vi "VI4.vi"() -> ()   [LabVIEW 2010]
panel:
  in  "AS_RS Ativado":bool
  in  "Elevar Z":bool
  in  "ARMAZEM_PEGAR":bool
  in  "ESTEIRA_PEGAR":bool
  out "YD3":dbl
  out "YD2":dbl
  out "YD1":dbl
  out "YD0":dbl
  in  "Coordenada_Y":dbl min=0.0 max=2.0
  out "Z_Pos_Ok":bool
  out "Y_Pos_Ok":bool
  out "X_Pos_Ok":bool
  out "Z_Home_Ok":bool
  out "Y_Home_Ok":bool
  out "X_Home_Ok":bool
  in  "Z_CTRG":bool
  in  "Y_CTRG":bool
  in  "X_CTRG":bool
  in  "Z_HOME":bool
  in  "Y_HOME":bool
  in  "X_HOME":bool
  in  "Start":bool
  in  "Confirmação da posição":bool
  out "ZD3":dbl
  out "ZD2":dbl
  out "ZD1":dbl
  out "ZD0":dbl
  out "XD3":dbl
  out "XD2":dbl
  out "XD1":dbl
  out "XD0":dbl
  in  "Coordenada_Z":dbl min=0.0 max=12.0
  in  "Coordenada_X":dbl min=0.0 max=6.0
  out "Esteira 4":bool
  out "Esteira 3":bool
  out "Esteira 2":bool
  out "Esteira 1":bool
  in  "Eletroválvula 4":bool
  in  "Eletroválvula 3":bool
  in  "Eletroválvula 2":bool
  in  "Eletroválvula 1":bool
  out "Sensor 4":bool
  out "Sensor 3":bool
  out "Sensor 2":bool
  out "Sensor 1":bool
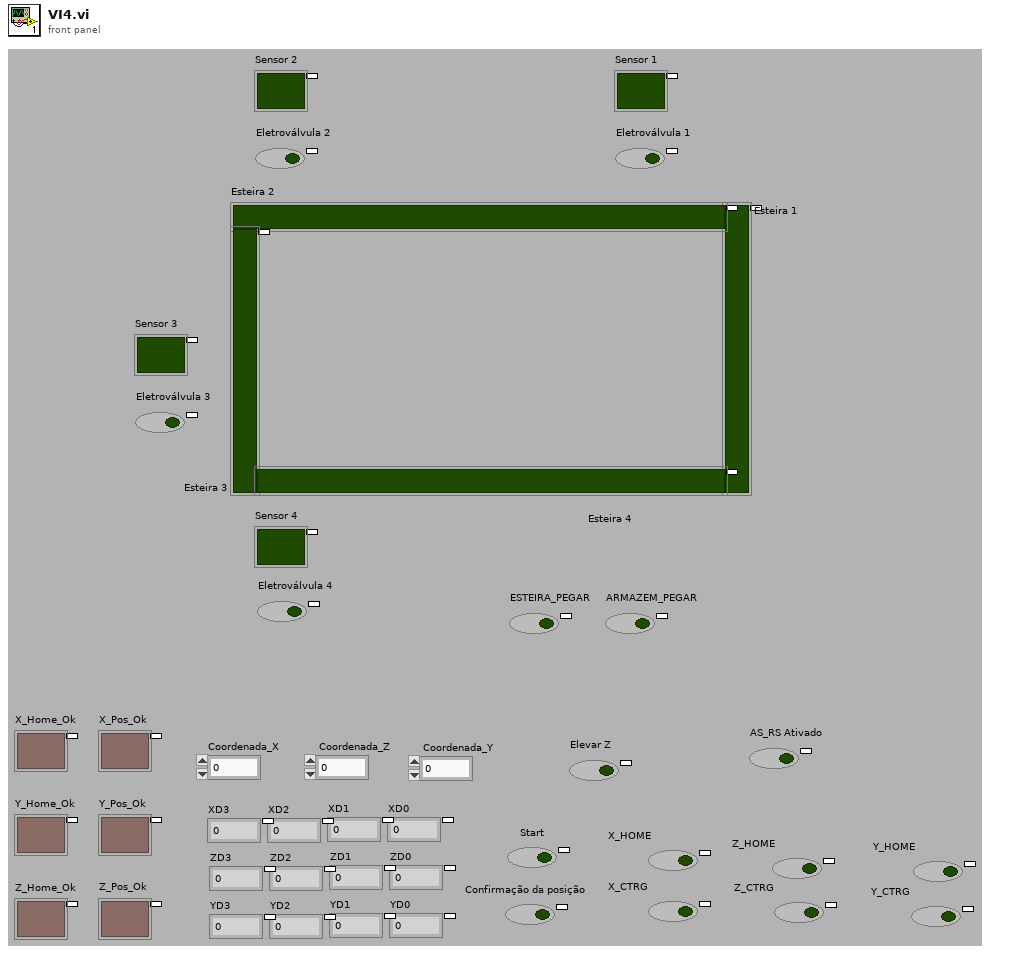
[diagram p1: front panel]
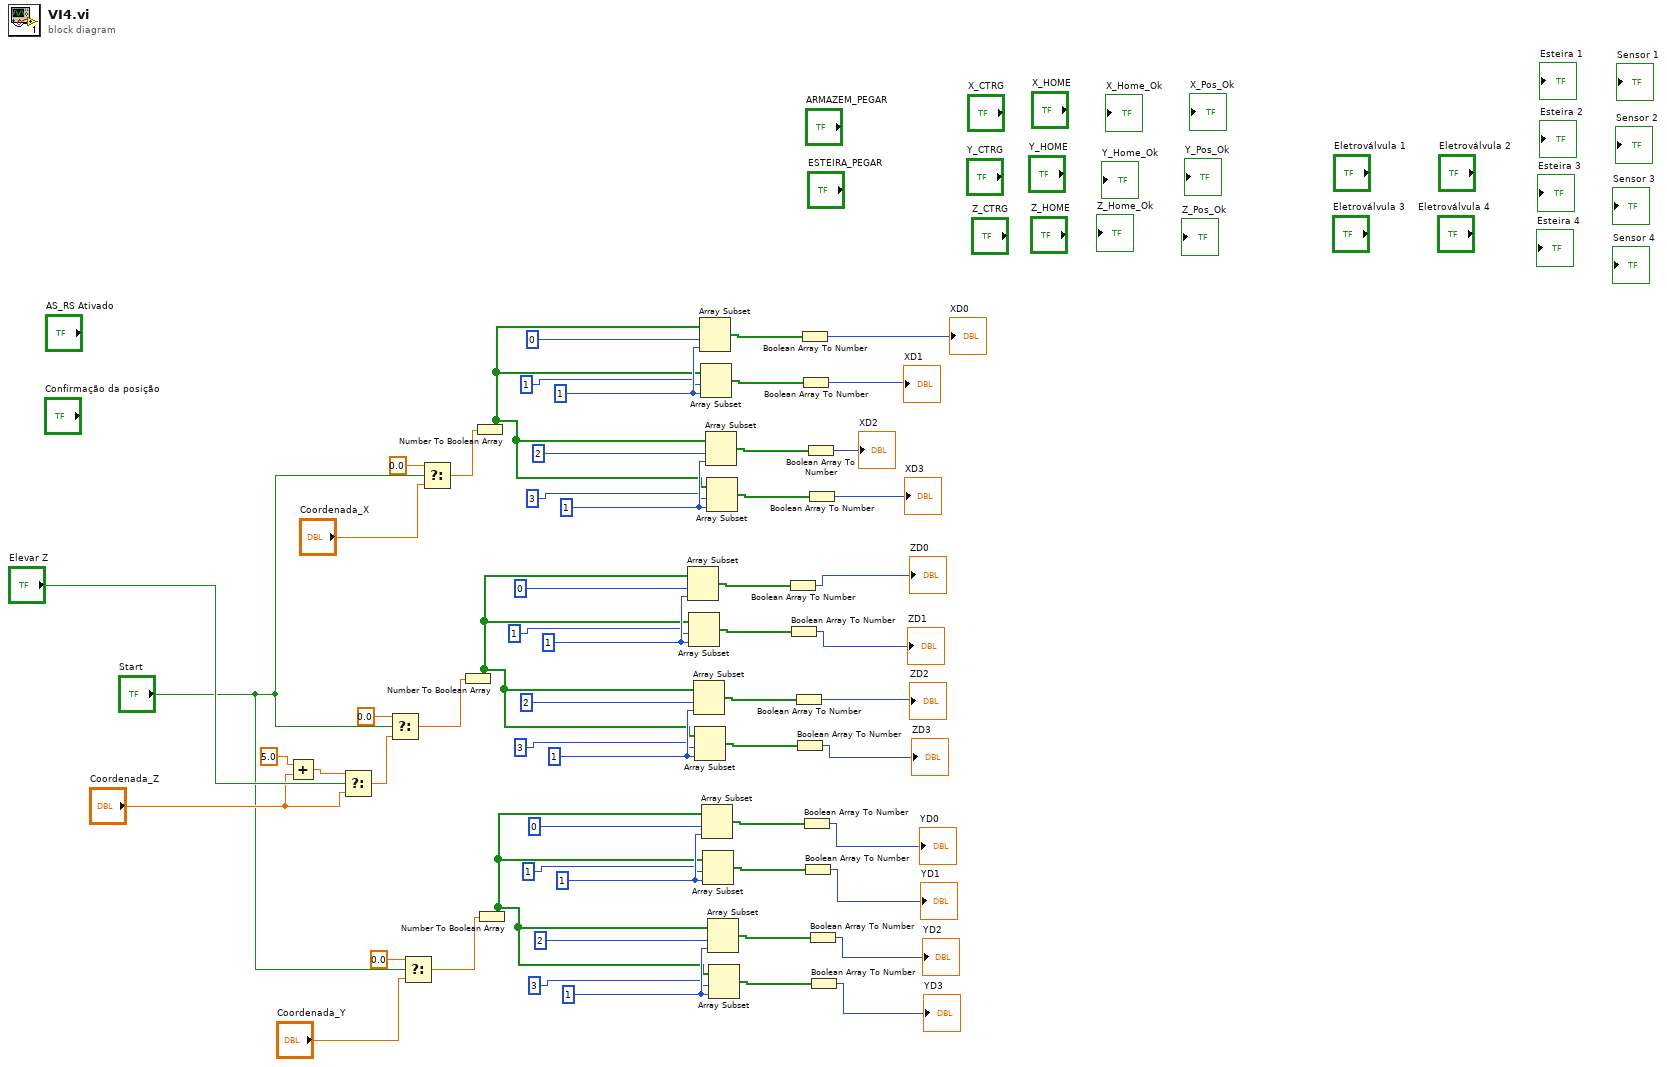
[diagram p0: block diagram]
diagram:
  w21 = 1 ("index")
  w26 = 1 ("index")
  w36 = 1 ("index")
  w41 = 1 ("index")
  w51 = 1 ("index")
  w56 = 1 ("index")
  n1 = Add(x=5.0, y="Coordenada_Z") -> (x+y=w3:dbl)
  n2 = Select(t=w3, s="Elevar Z", f="Coordenada_Z") -> (s? t:f=w2:dbl)
  n3 = Select(t=0.0, s="Start", f=w2) -> (s? t:f=w9:dbl)
  n4 = Select(t=0.0, s="Start", f="Coordenada_Y") -> (s? t:f=w7:dbl)
  n5 = Select(t=0.0, s="Start", f="Coordenada_X") -> (s? t:f=w11:dbl)
  n6 = Number To Boolean Array(number=w9) -> (Boolean array=w34:bool[])
  n7 = Number To Boolean Array(number=w11) -> (Boolean array=w49:bool[])
  n8 = Number To Boolean Array(number=w7) -> (Boolean array=w19:bool[])
  n9 = Array Subset(array=w34, index=0, length=w41) -> (w44:bool[])
  n10 = Array Subset(array=w34, index=1, length=w41) -> (w42:bool[])
  n11 = Array Subset(array=w34, index=2, length=w36) -> (w39:bool[])
  n12 = Array Subset(array=w34, index=3, length=w36) -> (w37:bool[])
  n13 = Array Subset(array=w49, index=0, length=w56) -> (w59:bool[])
  n14 = Array Subset(array=w49, index=1, length=w56) -> (w57:bool[])
  n15 = Array Subset(array=w19, index=0, length=w26) -> (w29:bool[])
  n16 = Array Subset(array=w19, index=1, length=w26) -> (w27:bool[])
  n17 = Array Subset(array=w49, index=2, length=w51) -> (w54:bool[])
  n18 = Array Subset(array=w49, index=3, length=w51) -> (w52:bool[])
  n19 = Array Subset(array=w19, index=2, length=w21) -> (w24:bool[])
  n20 = Array Subset(array=w19, index=3, length=w21) -> (w22:bool[])
  n21 = Boolean Array To Number(Boolean array=w44) -> (number=→"ZD0":u32)
  n22 = Boolean Array To Number(Boolean array=w42) -> (number=→"ZD1":u32)
  n23 = Boolean Array To Number(Boolean array=w39) -> (number=→"ZD2":u32)
  n24 = Boolean Array To Number(Boolean array=w37) -> (number=→"ZD3":u32)
  n25 = Boolean Array To Number(Boolean array=w59) -> (number=→"XD0":u32)
  n26 = Boolean Array To Number(Boolean array=w57) -> (number=→"XD1":u32)
  n27 = Boolean Array To Number(Boolean array=w29) -> (number=→"YD0":u32)
  n28 = Boolean Array To Number(Boolean array=w27) -> (number=→"YD1":u32)
  n29 = Boolean Array To Number(Boolean array=w54) -> (number=→"XD2":u32)
  n30 = Boolean Array To Number(Boolean array=w52) -> (number=→"XD3":u32)
  n31 = Boolean Array To Number(Boolean array=w24) -> (number=→"YD2":u32)
  n32 = Boolean Array To Number(Boolean array=w22) -> (number=→"YD3":u32)
